vi "_PC_SaveFile spectrumAsMAT.vi"(7 "path refnum in":refnum<file>, 8 "error in (no error)":errorcluster, 10 "Spectrum data in":waveform(sgl)) -> (0 "error out":errorcluster)   [LabVIEW 2018]
uses:
  PublicSubVI/Class/Sig2MS/Sig2MS.lvclass
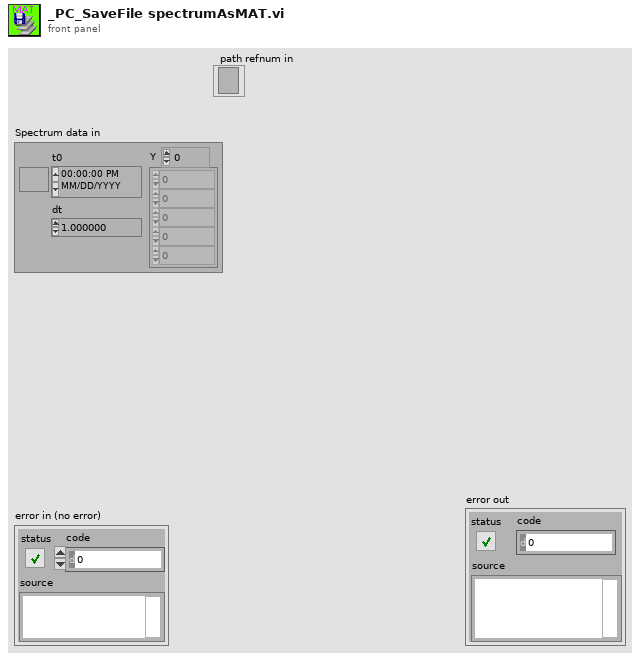
[diagram p1: front panel]
types:
  T1 = enum16{"init", "loadScript", "newScript", "runScript", "close"}
  T2 = cluster{"startTime":dbl, "scanSig":cluster{"priDt":dbl, "priXData":dbl[], "priYData":sgl[], "beta":dbl[]}[], "ionSig":cluster{"secDt":dbl, "secYData":sgl[]}[]}
  T3 = cluster{"startTime":dbl, "scanData":cluster{"dt":dbl, "xdata":dbl[], "ydata":sgl[], "beta":dbl[]}[], "xyXLabel":string, "xyYLabel":string, "wfmXLabel":string, "wfmYLabel":string, "ionData":cluster{"dt":dbl, "ydata":sgl[]}[], "ionXLabel":string, "ionYLabel":string}
  T4 = cluster{"dt":dbl, "xdata":dbl[], "ydata":sgl[], "beta":dbl[]}[]
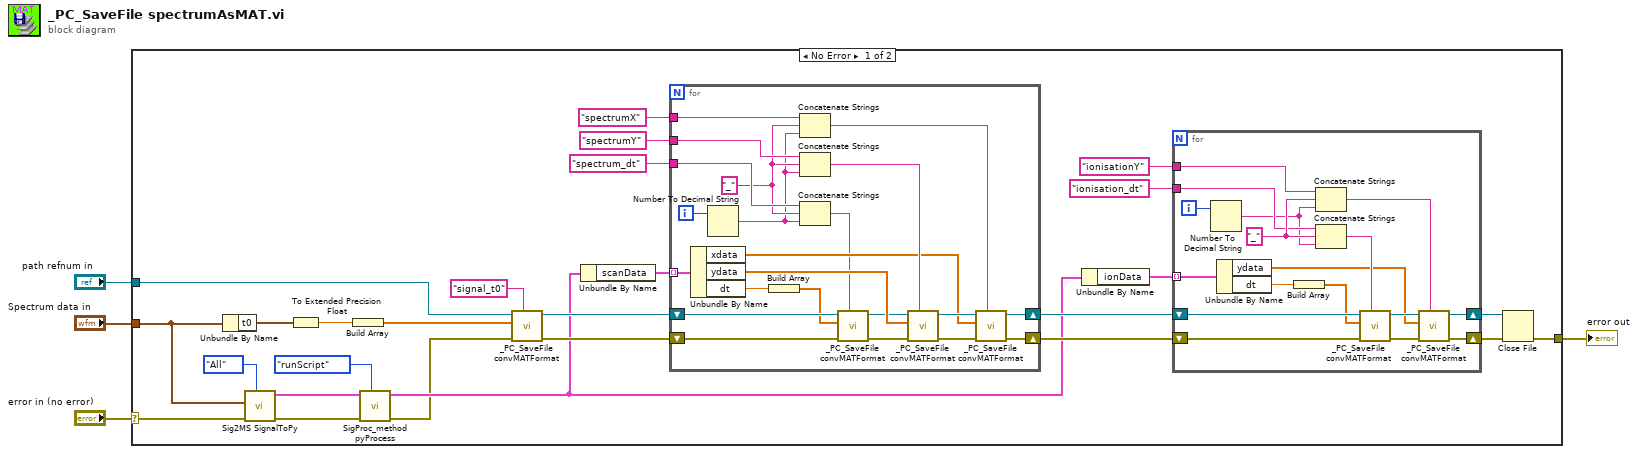
[diagram p0: block diagram]
diagram:
  n1 = case shown="No Error" "error in (no error)" {
    selector: "error in (no error)" -> [w7 w71]
    tunnel: [w31 w71] -> w4
    tunnel: "Spectrum data in" -> [w13 _]
    tunnel: "path refnum in" -> [w5 _]
    frame No Error {
      n2 = Unbundle By Name(w13) -> ("t0"=w30:timestamp)
      n3 = call "Sig2MS SignalToPy.vi"("getType"=enum16{"All", "Spectra", "Ionisation"}."All", "error in (no error)"=w7, "rawSignal"=w13) -> ("error out"=w15:errorcluster, "pySigFormat"=w16:T2)  [unwired: 7 in]
      n4 = To Extended Precision Float(1:w30) -> (0:w26:ext)
      n5 = Build Array(w26) -> (w25:ext[])
      n6 = call "SigProc_method pyProcess.vi"("func"=T1."runScript", "error in (no error)"=w15, "dataParam"=w16) -> ("error out"=w6:errorcluster, "newSigInfo"=w10:T3)  [unwired: 5 in, 2 out]
      n7 = call "_PC_SaveFile convMATFormat.vi"("Matrix Name"="signal_t0", "error in (no error)"=w6, "Data Array"=w25, "path refnum in"=w5) -> ("error out"=w24:errorcluster, "path refnum out"=w23:refnum<file>)  [unwired: 6 in]
      n8 = Unbundle By Name(w10) -> ("scanData"=w12:T4)
      n9 = for {
        tunnel: "spectrumY" ("Matrix Name") -> [w64]
        tunnel: "spectrumX" ("Matrix Name") -> [w62]
        shift-right: [w67] -> w21
        shift-left: w24 -> [w54]
        shift-right: [w68] -> w22
        shift-left: w23 -> [w55]
        tunnel: w12 -> [w66] mode=indexing
        tunnel: "spectrum_dt" ("Matrix Name") -> [w58]
        i -> [w65]
        w57 = "_" ("string")
        n10 = Unbundle By Name(w66) -> ("xdata"=w60:dbl[], "ydata"=w59:sgl[], "dt"=w51:dbl)
        n11 = Number To Decimal String(number=w65) -> (decimal integer string=w56:string)  [unwired: 1 in]
        n12 = Build Array(w51) -> (w50:dbl[])
        n13 = Concatenate Strings(w62, w57, w56) -> (w61:string)
        n14 = Concatenate Strings(w64, w57, w56) -> (w63:string)
        n15 = Concatenate Strings(w58, w57, w56) -> (w49:string)
        n16 = call "_PC_SaveFile convMATFormat.vi"("Matrix Name"=w49, "error in (no error)"=w54, "Data Array"=w50, "path refnum in"=w55) -> ("error out"=w53:errorcluster, "path refnum out"=w52:refnum<file>)  [unwired: 6 in]
        n17 = call "_PC_SaveFile convMATFormat.vi"("Matrix Name"=w63, "error in (no error)"=w53, "Data Array"=w59, "path refnum in"=w52) -> ("error out"=w69:errorcluster, "path refnum out"=w70:refnum<file>)  [unwired: 6 in]
        n18 = call "_PC_SaveFile convMATFormat.vi"("Matrix Name"=w61, "error in (no error)"=w69, "Data Array"=w60, "path refnum in"=w70) -> ("error out"=w67:errorcluster, "path refnum out"=w68:refnum<file>)  [unwired: 6 in]
      }
      n19 = Unbundle By Name(w10) -> ("ionData"=w9:cluster{"dt":dbl, "ydata":sgl[]}[])
      n20 = for {
        shift-right: [w40] -> w17
        shift-left: w21 -> [w34]
        shift-right: [w41] -> w18
        shift-left: w22 -> [w35]
        tunnel: "ionisationY" ("Matrix Name") -> [w45]
        tunnel: "ionisation_dt" ("Matrix Name") -> [w44]
        tunnel: w9 -> [w38] mode=indexing
        i -> [w48]
        w46 = "_" ("string")
        n21 = Number To Decimal String(number=w48) -> (decimal integer string=w36:string)  [unwired: 1 in]
        n22 = Unbundle By Name(w38) -> ("ydata"=w32:sgl[], "dt"=w37:dbl)
        n23 = Build Array(w37) -> (w33:dbl[])
        n24 = Concatenate Strings(w45, w46, w36) -> (w39:string)
        n25 = Concatenate Strings(w44, w46, w36) -> (w47:string)
        n26 = call "_PC_SaveFile convMATFormat.vi"("Matrix Name"=w47, "error in (no error)"=w34, "Data Array"=w33, "path refnum in"=w35) -> ("error out"=w42:errorcluster, "path refnum out"=w43:refnum<file>)  [unwired: 6 in]
        n27 = call "_PC_SaveFile convMATFormat.vi"("Matrix Name"=w39, "error in (no error)"=w42, "Data Array"=w32, "path refnum in"=w43) -> ("error out"=w40:errorcluster, "path refnum out"=w41:refnum<file>)  [unwired: 6 in]
      }
      n28 = Close File(refnum=w18, error in=w17) -> (error out=w31:errorcluster)  [unwired: 1 out]
    }
    frame Error {
    }
  }
  "error out" <- w4
